vi "Read-Save DefaultNotes.vi"(6 "Task":enum16{"Save", "Read"}(ring)=enum."Read", 11 "Notes":string) -> (0 "Pref Path":path, 3 "Notes Out":string)   [LabVIEW 2022 SP3]
panel:
  out "text":string
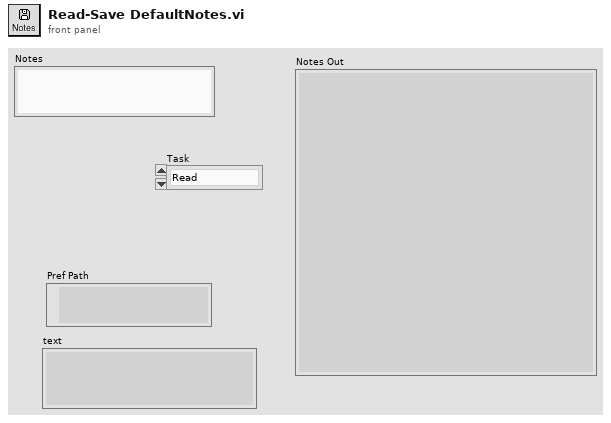
[diagram p1: front panel]
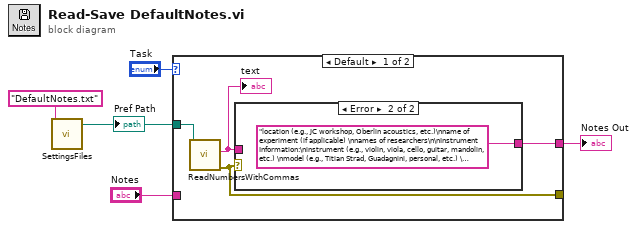
[diagram p0: block diagram]
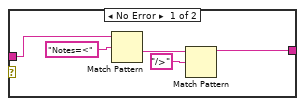
[diagram p2: hidden frame]
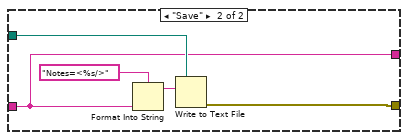
[diagram p3: hidden frame]
diagram:
  n1 = call "SettingsFiles.vi"("settings file name"="DefaultNotes.txt" ("name or relative path")) -> ("file path"=w1:path)  [unwired: 9 in, 1 out]
  "Pref Path" <- w1
  n2 = case shown="Default" "Task" {
    tunnel: "Notes" -> [_ w16]
    tunnel: w1 -> [w8 w20]
    tunnel: [w6 w17] -> _
    tunnel: [w9 w16] -> w3
    frame Default {
      n3 = call "ReadNumbersWithCommas.vi"("file (use dialog)"=w8) -> ("error out"=w6:errorcluster, "text"=w7:string)  [unwired: 7 in, 2 out]
      "text" <- w7
      n4 = case shown="Error" w6 {
        tunnel: [w10 "location (e.g., JC workshop, Oberlin acoustics, etc.)\nname of experiment (if applicable) \nnames of researchers\n\nInstrument Information:\ninstrument (e.g., violin, viola, cello, guitar, mandolin, etc.) \nmodel (e.g., Titian Strad, Guadagnini, personal, etc.) \nmaker name\nmaker ID (e.g., serial number)\nyear built (4 digits)\ncountry of origin \nsession (e.g. Oberlin 2017, VSA 2008) \nmaking school (e.g. Old Italian) \n\nMeasurement Information:\ntype (Radiation, admittance, modal analysis, taptones, etc.) \nprotocol (HV24, etc.)\n" ("Notes")] -> w9
        tunnel: w7 -> [w14 _]
        frame No Error {
          n5 = Match Pattern(string=w14, regular expression="Notes=<" ("format string")) -> (after substring=w13:string)  [unwired: 1 in, 3 out]
          n6 = Match Pattern(string=w13, regular expression="/>" ("format string")) -> (before substring=w10:string)  [unwired: 1 in, 3 out]
        }
        frame Error {
        }
      }
    }
    frame "Save" {
      n7 = Format Into String(format string="Notes=<%s/>", w16) -> (resulting string=w19:string)  [unwired: 2 in, 1 out]
      n8 = Write to Text File(file (use dialog)=w20, text=w19) -> (error out=w17:errorcluster)  [unwired: 2 in, 2 out]
    }
  }
  "Notes Out" <- w3
